vi "Get_Index_(X,Y)_from_TrackDot-2.vi"(2 "error IN":errorcluster, 3 "# frame\nof dot":i32, 4 "[IN] Dot":cluster{"X":dbl, "Y":dbl, "dX":dbl, "dY":dbl}, 5 "[IN] X,Y":dbl[][](array[numeric])) -> (0 "error OUT":errorcluster, 1 "Index in column\nof dot for AREA":i32)   [LabVIEW 2013]
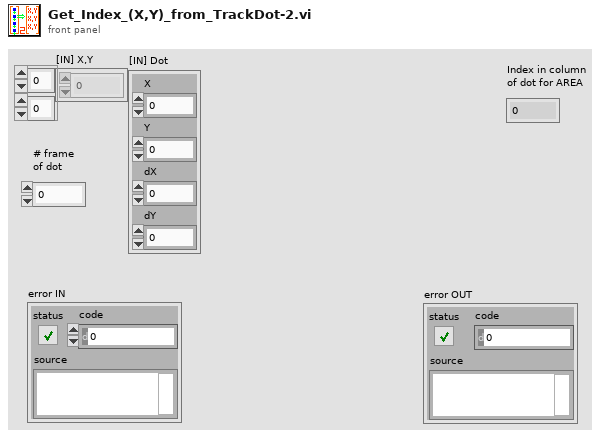
[diagram p1: front panel]
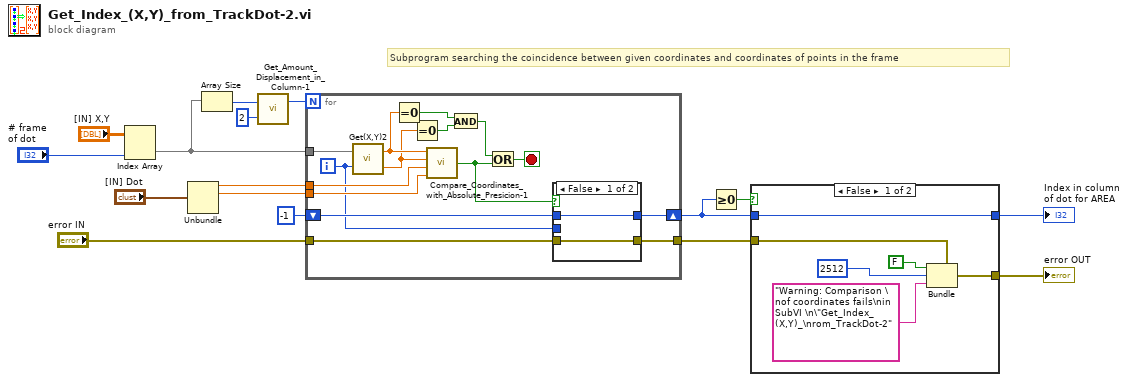
[diagram p0: block diagram]
diagram:
  # "Subprogram searching the coincidence between given coordinates and coordinates of points in the frame"
  n1 = Index Array(array="[IN] X,Y", index (col)="# frame\nof dot") -> (element=w6:dbl[])  [unwired: 1 in]
  n2 = Unbundle("[IN] Dot") -> ("X"=w5:dbl, "Y"=w4:dbl)  [unwired: 2 out]
  n3 = Array Size(array=w6) -> (size(s)=w13:i32)
  n4 = call "Get_Amount_Displacement_in_Column-1.vi"("multiplier"=2, "# Rows"=w13) -> ("Displ amount"=w11:i32)  [unwired: 1 out]
  n5 = for {
    N: w11 -> [_]
    tunnel: w6 -> [w28]
    tunnel: w5 -> [w27]
    tunnel: w4 -> [w26]
    shift-right: [w30] -> w3
    shift-left: -1 -> [w19]
    tunnel: "error IN" -> [w17]
    tunnel: [w29] -> w7
    i -> [w18]
    stop <- w31 stop-if-true
    n6 = call "Get(X,Y)2.vi"("[IN] index of (X,Y)"=w18, "[IN] Array coordi\nnates (X,Y) in Frame"=w28) -> ("[OUT] Y"=w22:dbl, "[OUT] X"=w23:dbl)
    n7 = Equal To 0?(x=w23) -> (x = 0?=w25:bool)
    n8 = Equal To 0?(x=w22) -> (x = 0?=w24:bool)
    n9 = call "Compare_Coordinates_with_Absolute_Presicion-1.vi"("X 1"=w23, "Y 1"=w22, "X 2"=w27, "Y 2"=w26) -> ("[OUT] Same coordinates?"=w20:bool)  [unwired: 1 in]
    n10 = And(x=w25, y=w24) -> (x .and. y?=w21:bool)
    n11 = Or(x=w21, y=w20) -> (x .or. y?=w31:bool)
    n12 = case shown="False" w20 {
      tunnel: w17 -> [w32 w35]
      tunnel: w18 -> [_ w34]
      tunnel: w19 -> [w33 _]
      tunnel: [w32 w35] -> w29
      tunnel: [w33 w34] -> w30
      frame False {
      }
      frame True {
      }
    }
  }
  n13 = Greater Or Equal To 0?(x=w3) -> (x >= 0?=w9:bool)
  n14 = case shown="False" w9 {
    tunnel: w7 -> [w41 w42]
    tunnel: [w36 w42] -> w2
    tunnel: w3 -> [w37 w43]
    tunnel: [w37 w43] -> w1
    frame False {
      n15 = Bundle(cluster=w41, "status"=FALSE, "code"=2512, "source"="Warning: Comparison \nof coordinates fails\nin SubVI \n\"Get_Index_(X,Y)_\nrom_TrackDot-2") -> (w36:errorcluster)
    }
    frame True {
    }
  }
  "error OUT" <- w2
  "Index in column\nof dot for AREA" <- w1
